vi "GetButton.vi"(0 "reference in":refnum<class "Button.lvclass">, 5 "error in (no error)":errorcluster) -> (14 "reference out":refnum<class "Button.lvclass">, 19 "error out":errorcluster)   [LabVIEW 2019, in "Button.lvclass"]
doc: "Draws A button"
uses:
  Button.lvclass
  C:/Users/Taylor.Hillegeist/OneDrive - Ultra/LabVIEW/Pgui2/Pgui_Obj_class/Pgui_Obj.lvclass
  Pgui_Obj_class/Pgui_Obj.lvclass
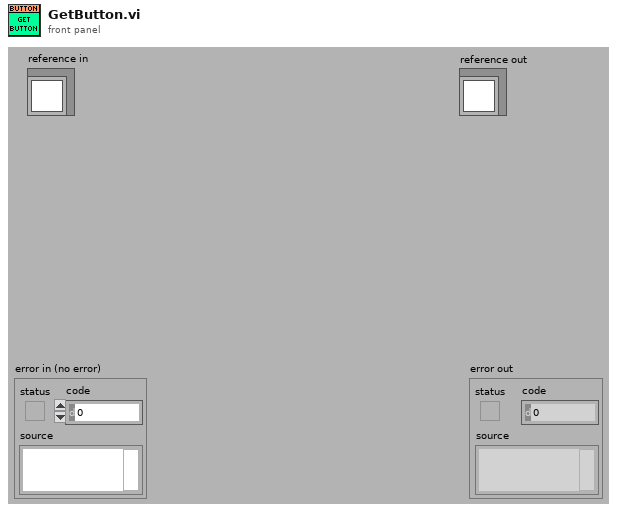
[diagram p1: front panel]
types:
  T1 = cluster{"horizontal":enum16{"left", "center", "right"}, "vertical":enum16{"top", "center", "bottom"}}
  T2 = cluster{"left":i16, "top":i16, "right":i16, "bottom":i16}
  T3 = typedef "Button.lvclass/ObjectAttributes.ctl" = cluster{"Text":string, "Override size":cluster{"Width":i16, "Height":i16}}
  T4 = typedef "Pgui_Obj.lvclass/ObjectAttributes.ctl" = cluster{"Children":refnum<class "Pgui_Obj.lvclass">[], "Draw Instr":picture, "Params":cluster{"left":i16, "top":i16, "right":i16, "bottom":i16}, "Parent_Pgui_Obj":refnum<class "Pgui_Obj.lvclass">, "MouseOver":bool}
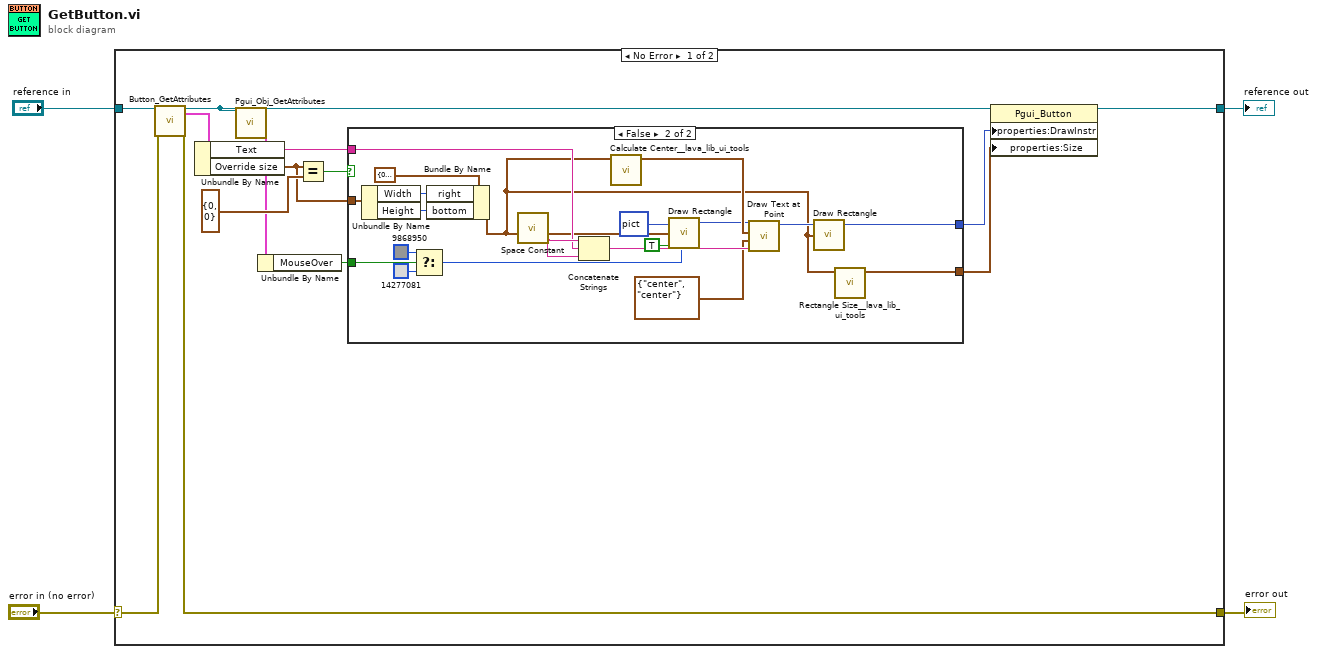
[diagram p0: block diagram]
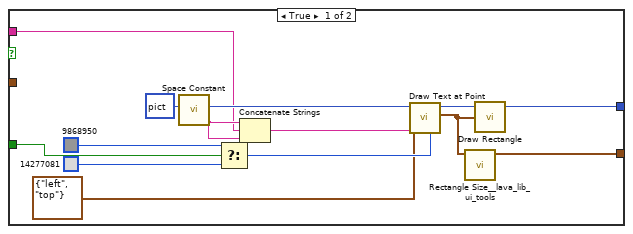
[diagram p2: hidden frame]
diagram:
  n1 = case shown="No Error" "error in (no error)" {
    selector: "error in (no error)" -> [w18 w53]
    tunnel: [w16 w53] -> w3
    tunnel: [w9 w52] -> w1
    tunnel: "reference in" -> [w15 w52]
    frame No Error {
      n2 = call "Button_GetAttributes.vi"("reference in"=w15, "error in (no error)"=w18) -> ("reference out"=w13:refnum<class "Button.lvclass">, "Data"=w17:T3, "error out"=w16:errorcluster)  [unwired: 14 in, 1 out]
      n3 = Unbundle By Name(w17) -> ("Text"=w10:string, "Override size"=w5:cluster{"Width":i16, "Height":i16})
      n4 = call "Pgui_Obj_GetAttributes.vi"("reference in"=w13) -> ("Data"=w12:T4)  [unwired: 15 in, 3 out]
      n5 = Unbundle By Name(w12) -> ("MouseOver"=w11:bool)
      n6 = Equal?(x=w5, y=cluster{"Width":i16, "Height":i16} {"Width"=0, "Height"=0}) -> (x = y?=w6:bool)
      n7 = case shown="False" w6 {
        tunnel: w11 -> [w23 w46]
        tunnel: w10 -> [w22 w45]
        tunnel: [w21 w44] -> w8
        tunnel: [w19 w43] -> w7
        tunnel: w5 -> [_ w38]
        frame True {
          n8 = call <vilib>:"Space Constant.vi"() -> ("String"=w31:string)
          n9 = Select(t=u32 9868950 ("BG color(transparent)"), s=w23, f=u32 14277081 ("BG color(transparent)")) -> (s? t:f=w27:u32)
          n10 = Concatenate Strings(w31, w22, w31) -> (w30:string)
          n11 = call <vilib>:"Draw Text at Point.vi"("BG color(transparent)"=w27, "text"=w30, "alignment(left, top)"=T1 {"horizontal"=enum."left", "vertical"=enum."top"}, "picture"=picture data[5B]) -> ("text rect"=w29:T2, "new picture"=w28:picture)  [unwired: 6 in]
          n12 = call <vilib>:"Rectangle Size__lava_lib_ui_tools.vi"("Rectangle"=w29) -> ("Rect Size"=w19:cluster{"width":i32, "height":i32})  [unwired: 8 in, 2 out]
          n13 = call <vilib>:"Draw Rectangle.vi"("picture"=w28, "rect"=w29) -> ("new picture"=w21:picture)  [unwired: 7 in]
        }
        frame False {
          n14 = Unbundle By Name(w38) -> ("Width"=w37:i16, "Height"=w36:i16)
          n15 = Select(t=u32 9868950 ("BG color(transparent)"), s=w46, f=u32 14277081 ("BG color(transparent)")) -> (s? t:f=w40:u32)
          n16 = Bundle By Name(cluster=T2 {"left"=0, "top"=0, "right"=0, "bottom"=0} ("rect"), "right"=w37, "bottom"=w36) -> (w32:T2)
          n17 = call <vilib>:"Space Constant.vi"() -> ("String"=w51:string)
          n18 = Concatenate Strings(w51, w45, w51) -> (w50:string)
          n19 = call <vilib>:"Calculate Center__lava_lib_ui_tools.vi"("Rectangle"=w32) -> ("Center"=w42:cluster{"x":i32, "y":i32})  [unwired: 10 in]
          n20 = call <vilib>:"Draw Rectangle.vi"("picture"=picture data[5B], "rect"=w32, "fill?(F)"=TRUE, "color(black)"=w40) -> ("new picture"=w34:picture)  [unwired: 5 in]
          n21 = call <vilib>:"Draw Text at Point.vi"("text"=w50, "alignment(left, top)"=T1 {"horizontal"=enum."center", "vertical"=enum."center"}, "origin"=w42, "picture"=w34) -> ("new picture"=w49:picture)  [unwired: 6 in, 1 out]
          n22 = call <vilib>:"Draw Rectangle.vi"("picture"=w49, "rect"=w32) -> ("new picture"=w44:picture)  [unwired: 7 in]
          n23 = call <vilib>:"Rectangle Size__lava_lib_ui_tools.vi"("Rectangle"=w32) -> ("Rect Size"=w43:cluster{"width":i32, "height":i32})  [unwired: 8 in, 2 out]
        }
      }
      n24 = property class="Pgui_Button"(reference=w13, "properties:DrawInstr"=w8, "properties:Size"=w7) -> (reference out=w9:refnum<class "Button.lvclass">)  [unwired: 1 in, 1 out]
    }
    frame Error {
    }
  }
  "error out" <- w3
  "reference out" <- w1
